vi "LVPortPumpPropertyUpdates.vi"(11 "pID":string) -> (3 "Updating Bound Control Infos":T1[](array[typedef]))   [LabVIEW 2017]
uses:
  LVPortControlBindingInfoType.ctl
  LVPortControlBindingDirectionEnum.ctl
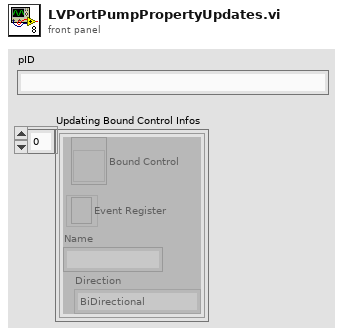
[diagram p1: front panel]
types:
  T1 = typedef "LVPortControlBindingInfoType.ctl" = cluster{"Bound Control":refnum<vi>, "Name":string, "Direction":T2, "Event Register":refnum<event-registration>}
  T2 = typedef "LVPortControlBindingDirectionEnum.ctl" = enum16{"BiDirectional", "ToMatlab", "ToLabview"}
  T3 = typedef "Dictionary Object RefNum__ogtk.ctl" = refnum<k1>
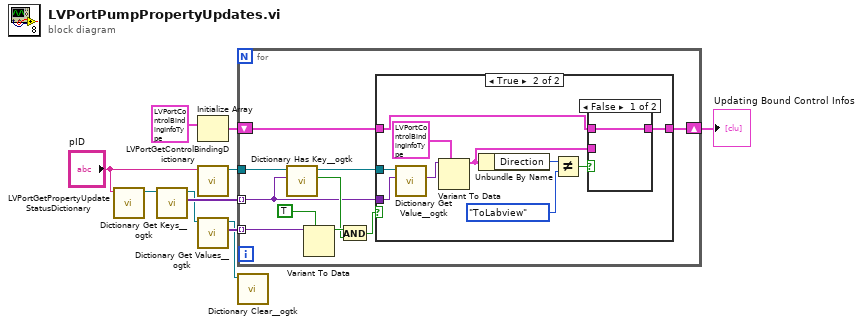
[diagram p0: block diagram]
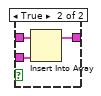
[diagram p3: hidden frame]
diagram:
  n1 = call "LVPortGetPropertyUpdateStatusDictionary.vi"("pID"="pID") -> ("Refnum out"=w10:T3)  [unwired: 10 in]
  n2 = call <userlib>:"Dictionary Get Keys__ogtk.vi"("dictionary"=w10) -> ("keys"=w8:variant[], "dictionary out"=w6:T3)  [unwired: 8 in, 1 out]
  n3 = Initialize Array(T1 {"Bound Control"=refnum, "Name"="", "Direction"=enum."BiDirectional", "Event Register"=refnum} ("Control Binding Info")) -> (w3:T1[])  [unwired: 1 in]
  n4 = call "LVPortGetControlBindingDictionary.vi"("pID"="pID") -> ("Refnum out"=w7:T3)  [unwired: 10 in]
  n5 = call <userlib>:"Dictionary Get Values__ogtk.vi"("dictionary"=w6) -> ("values"=w9:variant[], "dictionary out"=w5:T3)  [unwired: 8 in, 1 out]
  n6 = for {
    tunnel: w9 -> [w20] mode=indexing
    tunnel: w8 -> [w11] mode=indexing
    tunnel: w7 -> [w18]
    shift-right: [w12] -> w1
    shift-left: w3 -> [w13]
    n7 = call <userlib>:"Dictionary Has Key__ogtk.vi"("key"=w11, "dictionary"=w18) -> ("Has Key?"=w16:bool, "dictionary out"=w14:T3)  [unwired: 7 in, 1 out]
    n8 = Variant To Data(type=TRUE, Variant=w20) -> (data=w17:bool)  [unwired: 1 in, 1 out]
    n9 = And(x=w17, y=w16) -> (x .and. y?=w15:bool)
    n10 = case shown="True" w15 {
      tunnel: w14 -> [_ w28]
      tunnel: w13 -> [w21 w25]
      tunnel: [w21 w23] -> w12
      tunnel: w11 -> [_ w22]
      frame False {
      }
      frame True {
        n11 = call <userlib>:"Dictionary Get Value__ogtk.vi"("key"=w22, "dictionary"=w28) -> ("value"=w27:variant)  [unwired: 6 in, 3 out]
        n12 = Variant To Data(type=T1 {"Bound Control"=refnum, "Name"="", "Direction"=enum."BiDirectional", "Event Register"=refnum} ("Control Binding Info"), Variant=w27) -> (data=w24:T1)  [unwired: 1 in, 1 out]
        n13 = Unbundle By Name(w24) -> ("Direction"=w30:T2)
        n14 = Not Equal?(x=w30, y=LVPortControlBindingDirectionEnum."ToLabview") -> (x != y?=w26:bool)
        n15 = case shown="False" w26 {
          tunnel: w25 -> [w32 w35]
          tunnel: w24 -> [_ w34]
          tunnel: [w32 w33] -> w23
          frame False {
          }
          frame True {
            n16 = Insert Into Array(array=w35, new element=w34) -> (w33:T1[])  [unwired: 1 in]
          }
        }
      }
    }
  }
  "Updating Bound Control Infos" <- w1
  n17 = call <userlib>:"Dictionary Clear__ogtk.vi"("dictionary"=w5) -> ()  [unwired: 9 in, 2 out]
